vi "Netburner_WR.vi"(0 "VISA resource name (COM Port #)":refnum<visa-resource-name>="COM7", 1 "String to Send":string="+test", 2 "Mode (0)":i32, 3 "Error In (no error)":errorcluster, 4 "Wait (sec)":dbl=0.25) -> (6 "Error Out":errorcluster={"status"=FALSE, "code"=1073676294, "source"="VISA Read in Galvant_GPIB_Sample.vi"})   [LabVIEW 2013]
uses:
  <vilib>/Instr/_visa.llb/VISA Configure Serial Port (Instr).vi
panel:
  out "Examples":string="Useful strings:\n+test\n+a:10\nID?"
  out "Number of Bytes sent":u32
  # "Netburner Write VI"
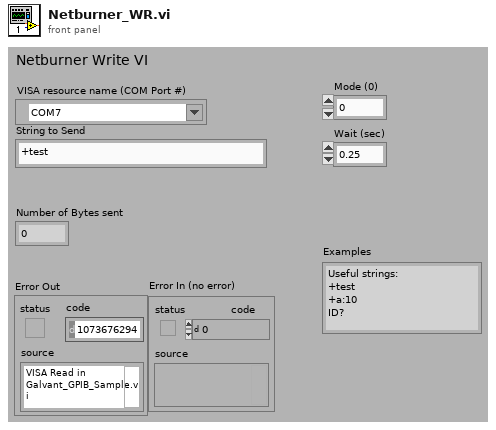
[diagram p1: front panel]
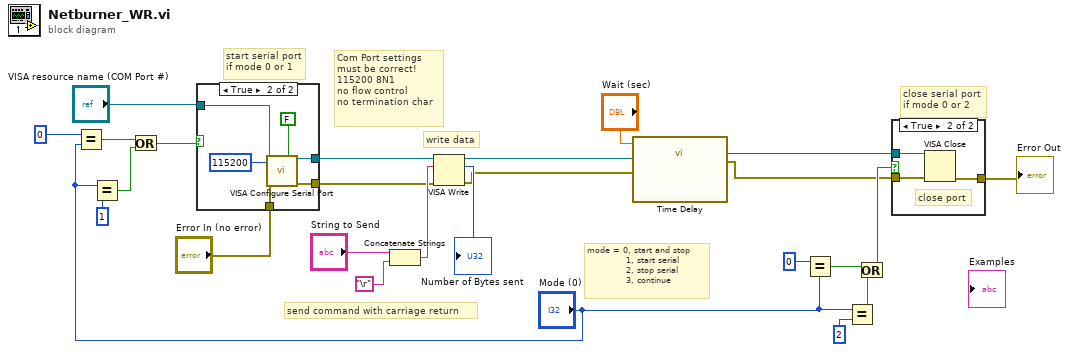
[diagram p0: block diagram]
diagram:
  # "write data"
  # "mode = 0, start and stop\n             1, start serial\n             2, stop serial\n             3, continue"
  # "Com Port settings\nmust be correct!\n115200 8N1\nno flow control\nno termination char"
  # "close serial port\nif mode 0 or 2"
  # "send command with carriage return"
  # "start serial port\nif mode 0 or 1"
  n1 = Equal?(x=0, y="Mode (0)") -> (x = y?=w9:bool)
  n2 = Equal?(x="Mode (0)", y=1) -> (x = y?=w7:bool)
  n3 = Or(x=w9, y=w7) -> (x .or. y?=w8:bool)
  n4 = case shown="True" w8 {
    tunnel: "VISA resource name (COM Port #)" -> [w26 w32]
    tunnel: [w26 w31] -> w19
    tunnel: [w25 w30] -> w18
    tunnel: "Error In (no error)" -> [w25 w27]
    frame False {
    }
    frame True {
      n5 = call-poly "VISA Configure Serial Port"("VISA resource name"=w32, "Enable Termination\nChar (T)"=FALSE, "baud rate (9600)"=115200, "error in (no error)"=w27) -> ("VISA resource name out"=w31:refnum<visa-resource-name>, "error out"=w30:errorcluster)  [unwired: 10 in]
    }
  }
  n6 = Concatenate Strings("String to Send", "\r") -> (w20:string)
  n7 = VISA Write(VISA resource name=w19, write buffer=w20, error in (no error)=w18) -> (VISA resource name out=w4:refnum<visa-resource-name>, return count=→"Number of Bytes sent":u32, error out=w3:errorcluster)
  n8 = call "Time Delay"("error in (no error)"=w3, "Delay Time (s)"="Wait (sec)") -> ("error out"=w2:errorcluster)  [unwired: 9 in]
  n9 = Equal?(x=0, y="Mode (0)") -> (x = y?=w13:bool)
  n10 = Equal?(x="Mode (0)", y=2) -> (x = y?=w11:bool)
  n11 = Or(x=w13, y=w11) -> (x .or. y?=w10:bool)
  n12 = case shown="True" w10 {
    tunnel: w4 -> [_ w36]
    tunnel: w2 -> [w33 w35]
    tunnel: [w33 w34] -> w23
    frame False {
    }
    frame True {
      # "close port"
      n13 = VISA Close(VISA resource name=w36, error in (no error)=w35) -> (error out=w34:errorcluster)
    }
  }
  "Error Out" <- w23
